vi "Serial InitMarvin.vi"(8 "error in (no error)":errorcluster, 9 "VI reference (current VI)":refnum<vi>, 11 "VISA Refnum in":refnum<visa-resource-name>) -> (0 "error out":errorcluster, 3 "Boolean":bool)   [LabVIEW 2017]
uses:
  <vilib>/Instr/_visa.llb/VISA Configure Serial Port (Instr).vi
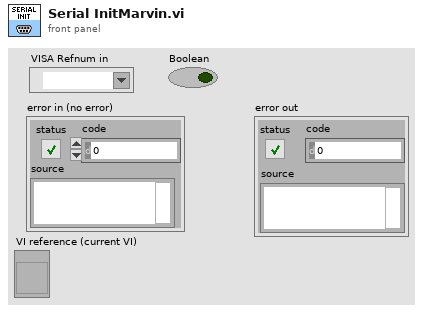
[diagram p1: front panel]
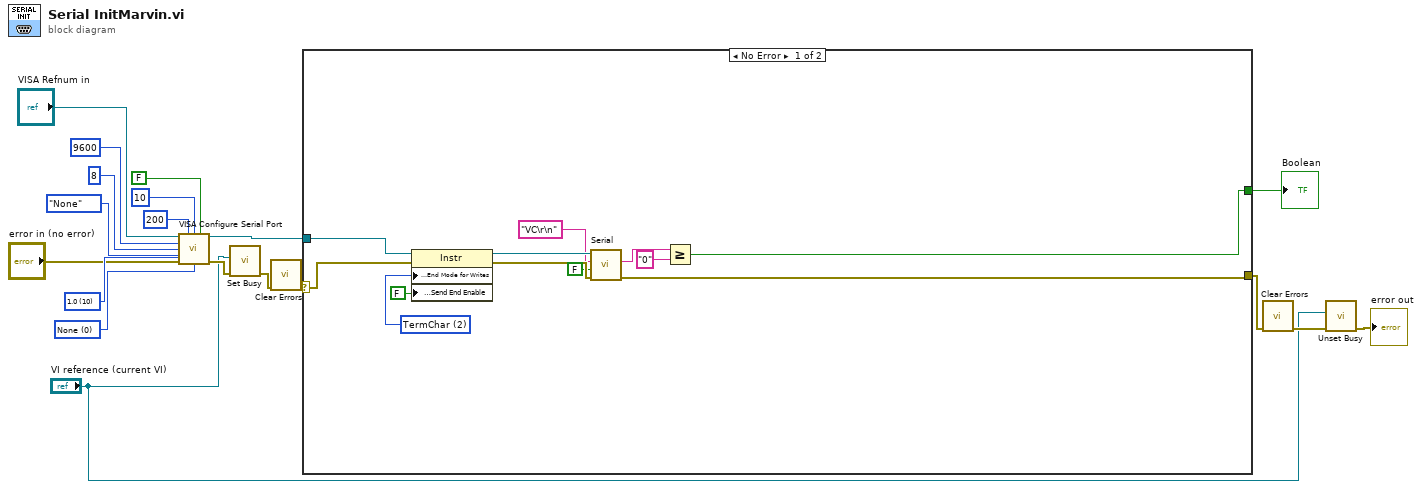
[diagram p0: block diagram]
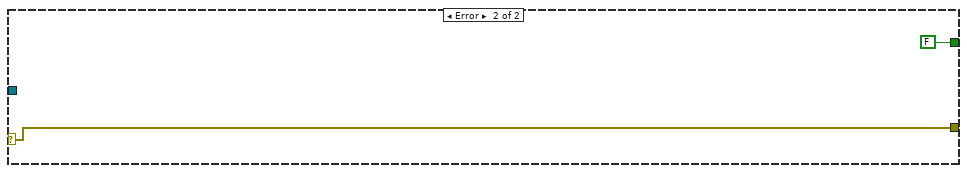
[diagram p2: hidden frame]
diagram:
  w16 = u16 0 items=["None", "XON/XOFF", "RTS/CTS", "XON/XOFF & RTS/CTS", "DTR/DSR", "XON/XOFF & DTR/DSR"] ("flow control (0:none)")
  w15 = u16 10 items=["1.0"=10, "1.5"=15, "2.0"=20] ("stop bits (10: 1 bit)")
  n1 = call-poly "VISA Configure Serial Port"("VISA resource name"="VISA Refnum in", "timeout (10sec)"=u32 200, "termination char\n(0xA = '\\n' = LF)"=u8 10 ("termination char\n(0xA = '\\n' = LF)"), "Enable Termination\nChar (T)"=FALSE ("Enable Termination\nChar (T)"), "baud rate (9600)"=u32 9600, "data bits (8)"=u16 8, "parity (0:none)"=enum16{"None", "Odd", "Even", "Mark", "Space"}."None", "error in (no error)"="error in (no error)", "stop bits (10: 1 bit)"=w15, "flow control (0:none)"=w16) -> ("VISA resource name out"=w17:refnum<visa-resource-name>, "error out"=w6:errorcluster)  [unwired: 4 in]
  n2 = call <vilib>:"Set Busy.vi"("error in (no error)"=w6, "VI reference (current VI)"="VI reference (current VI)") -> ("error out"=w5:errorcluster)  [unwired: 8 in, 1 out]
  n3 = call <vilib>:"Clear Errors.vi"("error in (no error)"=w5) -> ("error out"=w1:errorcluster)  [unwired: 5 in, 1 out]
  n4 = case shown="No Error" w1 {
    selector: w1 -> [w30 w32]
    tunnel: w17 -> [w31 _]
    tunnel: [w25 w32] -> w7
    tunnel: [w22 FALSE] -> w8
    frame No Error {
      w28 = u16 2 items=["None", "LastBit", "TermChar", "Break"] ("Serial Settings:Serial End Mode for Writes")
      n5 = property class="Instr"(reference=w31, error in=w30, "Serial Settings:End Mode for Writes"=w28, "Message Based Settings:Send End Enable"=FALSE) -> (reference out=w26:refnum<visa-resource-name>, error out=w27:errorcluster)
      n6 = call "Serial.vi"("error in (no error)"=w27, "Clear Log"=FALSE, "write buffer"="VC\r\n", "VISA resource name"=w26) -> ("error out"=w25:errorcluster, "read buffer"=w24:string)  [unwired: 6 in]
      n7 = Greater Or Equal?(x=w24, y="0") -> (x >= y?=w22:bool)
    }
    frame Error {
    }
  }
  "Boolean" <- w8
  n8 = call <vilib>:"Clear Errors.vi"("error in (no error)"=w7) -> ("error out"=w4:errorcluster)  [unwired: 5 in, 1 out]
  n9 = call <vilib>:"Unset Busy.vi"("error in (no error)"=w4, "VI reference (current VI)"="VI reference (current VI)") -> ("error out"=→"error out":errorcluster)  [unwired: 9 in]
